vi "CAN Write Flush.vi"(8 "error in (no error)":errorcluster, 11 "NI-XNET in":refnum<class "NI-XNET.lvclass">) -> (0 "error out":errorcluster, 3 "NI-XNET out":refnum<class "NI-XNET.lvclass">)   [LabVIEW 2023, in "HardwareAbstractionLayer_LVOOP.lvlib" / "CAN HAL Lib.lvlib" / "NI-XNET.lvclass"]
uses:
  NI-XNET.lvclass
  NI-XNET.lvclass/NI-XNET.ctl
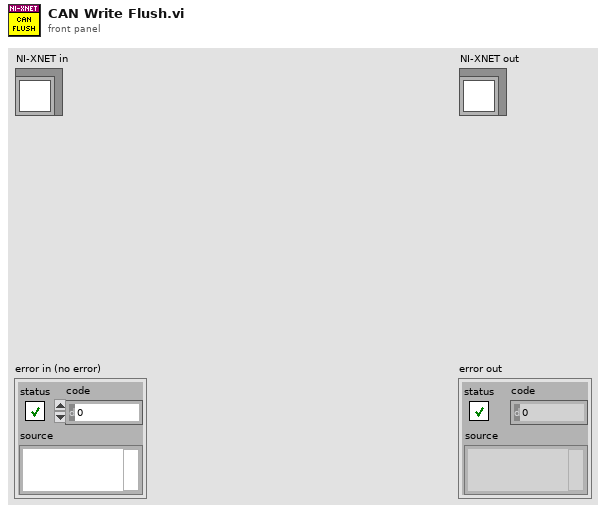
[diagram p1: front panel]
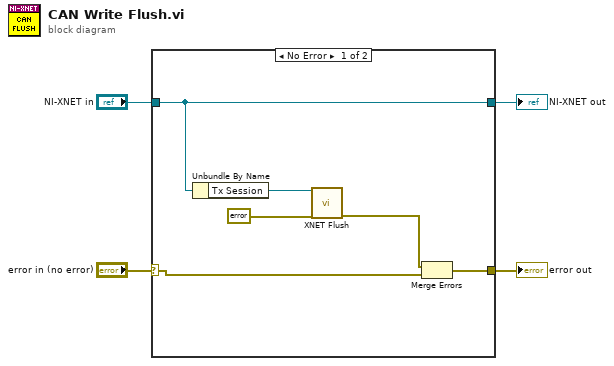
[diagram p0: block diagram]
diagram:
  n1 = case shown="No Error" "error in (no error)" {
    selector: "error in (no error)" -> [w6 w11]
    tunnel: [w7 w11] -> w3
    tunnel: "NI-XNET in" -> [w10 w12]
    tunnel: [w10 w12] -> w1
    frame No Error {
      n2 = Unbundle By Name(w10) -> ("Tx Session"=w9:refnum<k21>)
      n3 = call <vilib>:"XNET Flush.vi"("session in"=w9, "error in (no error)"=errorcluster {"status"=FALSE, "code"=0, "source"=""}) -> ("error out"=w8:errorcluster)  [unwired: 12 in, 1 out]
      n4 = Merge Errors(w8, w6) -> (w7:errorcluster)
    }
    frame Error {
    }
  }
  "error out" <- w3
  "NI-XNET out" <- w1
